vi "8164B GetInfo.vi"(8 "error in":errorcluster, 11 "KeySight 8164B control in":T1) -> (0 "error out":errorcluster, 3 "KeySight 8164B control out":T1)   [LabVIEW 2018, in "KeySight 8164B LAN InstrLib.lvlib"]
uses:
  KeySight 8164B LAN InstrLib.lvlib
  typedefs/KeySight 8164B control.ctl
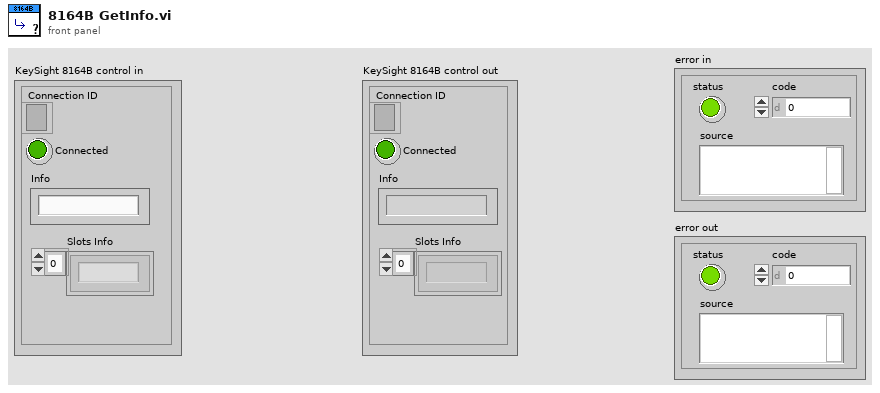
[diagram p1: front panel]
types:
  T1 = typedef "KeySight 8164B LAN InstrLib.lvlib/KeySight 8164B control.ctl" = cluster{"Connection ID":refnum<k5>, "Connected":bool, "Info":string, "Slots Info":string[]}
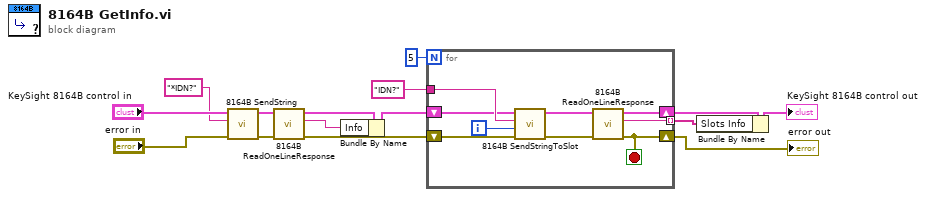
[diagram p0: block diagram]
diagram:
  n1 = call "8164B SendString.vi"("error in"="error in", "CMD"="*IDN?", "KeySight 8164B control in"="KeySight 8164B control in") -> ("error out"=w12:errorcluster, "KeySight 8164B control out"=w13:T1)  [unwired: 7 in]
  n2 = call "8164B ReadOneLineResponse.vi"("error in"=w12, "KeySight 8164B control in"=w13) -> ("error out"=w7:errorcluster, "OneLineResponse"=w11:string, "KeySight 8164B control out"=w9:T1)  [unwired: 7 in]
  n3 = Bundle By Name(cluster=w9, "Info"=w11) -> (w2:T1)
  n4 = for {
    N: 5 -> [_]
    tunnel: "IDN?" -> [w21]
    shift-right: [w22] -> w3
    shift-left: w7 -> [w20]
    shift-right: [w24] -> w6
    shift-left: w2 -> [w19]
    tunnel: [w23] -> w5 mode=indexing
    i -> [w16]
    stop <- w22 stop-if-true
    n5 = call "8164B SendStringToSlot.vi"("error in"=w20, "Slot Number"=w16, "CMD"=w21, "KeySight 8164B control in"=w19) -> ("error out"=w17:errorcluster, "KeySight 8164B control out"=w18:T1)  [unwired: 6 in]
    n6 = call "8164B ReadOneLineResponse.vi"("error in"=w17, "KeySight 8164B control in"=w18) -> ("error out"=w22:errorcluster, "OneLineResponse"=w23:string, "KeySight 8164B control out"=w24:T1)  [unwired: 7 in]
  }
  "error out" <- w3
  n7 = Bundle By Name(cluster=w6, "Slots Info"=w5) -> (→"KeySight 8164B control out":T1)
